vi "updateMMPayload.vi"(7 "path in":path=path "C:/dev/Hexagon-VTD-Custom-Device/Libraries/VC.dll", 8 "error in (no error)":errorcluster, 10 "payload":u8[](array[numeric]), 11 "mmHandle in":u64) -> (0 "error out":errorcluster, 1 "simFrame":dbl, 2 "simTime":dbl, 3 "mmHandle out":u64, 4 "return type":i32, 5 "isComplete":u8)   [LabVIEW 2023, in "MM.lvlib"]
uses:
  MM.lvlib
  RDB/RDB.lvlib
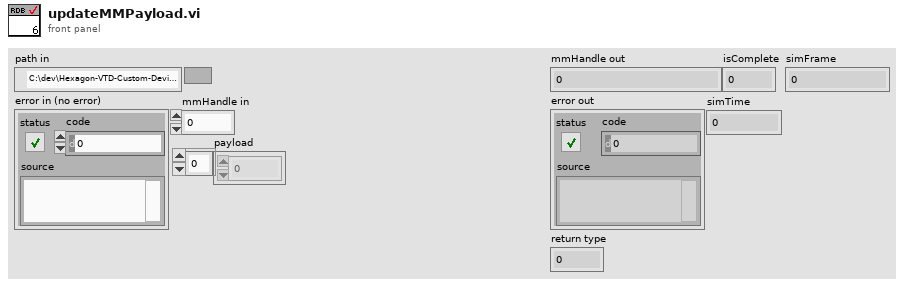
[diagram p1: front panel]
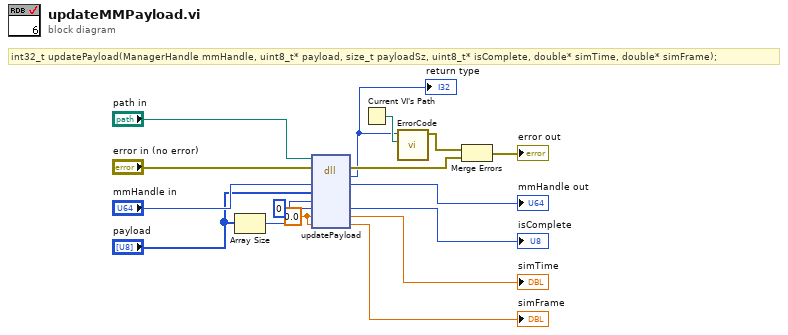
[diagram p0: block diagram]
diagram:
  w6 = 0.0 ("simTime")
  # "int32_t updatePayload(ManagerHandle mmHandle, uint8_t* payload, size_t payloadSz, uint8_t* isComplete, double* simTime, double* simFrame);"
  n1 = Array Size(array="payload") -> (size(s)=w8:i32)
  n2 = dll-call lib="C:/dev/Hexagon-VTD-Custom-Device/Libraries/libMM.dll" fn="updatePayload"(path in="path in", error in="error in (no error)", "mmHandle"="mmHandle in", "payload"="payload", "payloadSz"=w8, "isComplete"=u8 0, "simTime"=w6, "simFrame"=w6) -> (error out=w12:errorcluster, "return type"=w1:i32, "mmHandle"=→"mmHandle out":u64, "isComplete"=→"isComplete":u8, "simTime"=→"simTime":dbl, "simFrame"=→"simFrame":dbl)  [unwired: 3 in, 1 out]
  "return type" <- w1
  n3 = Current VI's Path() -> (path=w2:path)
  n4 = call "ErrorCode.vi"("parent VI path"=w2, "return type"=w1) -> ("error out"=w13:errorcluster)  [unwired: 9 in]
  n5 = Merge Errors(w13, w12) -> (→"error out":errorcluster)
